vi "Row and Col Num.vi"(7 "Option":T1, 8 "error in (no error)":errorcluster caption="错误输入（无错误）", 9 "NumCols In":u32, 10 "NumRow In":u32, 11 "Tree Class 输入":refnum<class "Tree Class.lvclass"> caption="DNL_LabVIEW Object in") -> (0 "error out":errorcluster caption="错误输出", 1 "NumCols Out":u32, 2 "NumRows Out":u32, 3 "Tree Class 输出":refnum<class "Tree Class.lvclass"> caption="DNL_LabVIEW Object out")   [LabVIEW 2012, in "Tree Tools.lvlib" / "Tree Class.lvclass"]
uses:
  Tree Class.lvclass
  Set Or Get Option.ctl
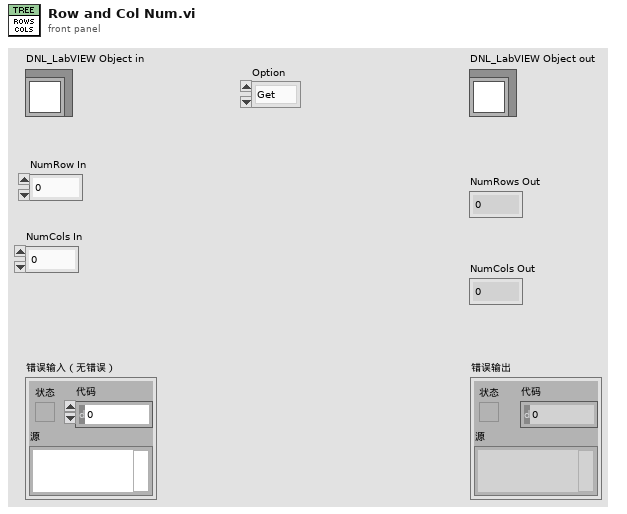
[diagram p1: front panel]
types:
  T1 = typedef "Tree Tools.lvlib/Tree Class.lvclass/Set Or Get Option.ctl" = enum16{"Get", "Set"}
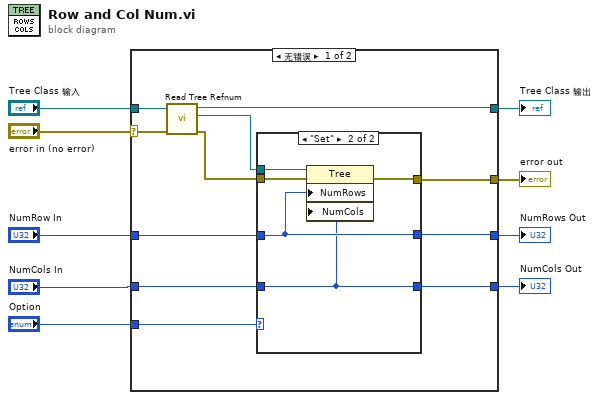
[diagram p0: block diagram]
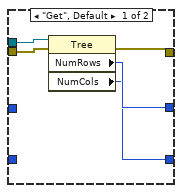
[diagram p2: hidden frame]
diagram:
  n1 = case shown="无错误" "error in (no error)" {
    selector: "error in (no error)" -> [w14 w32]
    tunnel: [w13 w32] -> w8
    tunnel: [w19 w31] -> w6
    tunnel: "Tree Class 输入" -> [w20 w31]
    tunnel: [w16 _] -> w5
    tunnel: [w15 _] -> w4
    tunnel: "NumRow In" -> [w12 _]
    tunnel: "NumCols In" -> [w11 _]
    tunnel: "Option" -> [w10 _]
    frame No Error {
      n2 = call-dynamic "Read Tree Refnum.vi"("error in (no error)"=w14, "Tree_LVOOP__lava_lib_tree_class in"=w20) -> ("error out"=w18:errorcluster, "Tree Refnum"=w17:refnum<vi>, "Tree_LVOOP__lava_lib_tree_class out"=w19:refnum<class "Tree Class.lvclass">)  [unwired: 7 in]
      n3 = case shown="\"Set\"" w10 {
        tunnel: w18 -> [w25 w30]
        tunnel: w17 -> [w24 w29]
        tunnel: [w23 w27] -> w16
        tunnel: [w22 w26] -> w15
        tunnel: [w21 w28] -> w13
        tunnel: w12 -> [_ w27]
        tunnel: w11 -> [_ w26]
        frame "Get", Default {
          n4 = property class="Tree"(reference=w24, error in=w25) -> (error out=w21:errorcluster, "NumRows"=w23:u32, "NumCols"=w22:u32)  [unwired: 1 out]
        }
        frame "Set" {
          n5 = property class="Tree"(reference=w29, error in=w30, "NumRows"=w27, "NumCols"=w26) -> (error out=w28:errorcluster)  [unwired: 1 out]
        }
      }
    }
    frame Error {
    }
  }
  "error out" <- w8
  "Tree Class 输出" <- w6
  "NumRows Out" <- w5
  "NumCols Out" <- w4
